vi "Utility Generate Instrument Error.vi"(8 "Error In":errorcluster, 9 "Code (0)":i32 format="%.0x", 10 "Status (F: No error)":bool, 11 "VISA Resource Name":refnum<visa-resource-name>) -> (0 "Error Out":errorcluster, 3 "VISA Resource Name Out":refnum<visa-resource-name>)   [LabVIEW 2010, in "Stanford Research 844.lvlib"]
doc: "This VI generates the error cluster with Error Code as code and chain of VI as source. The source does not include the name of this VI."
uses:
  <instrlib>/Stanford Research 844/Stanford Research 844.lvlib
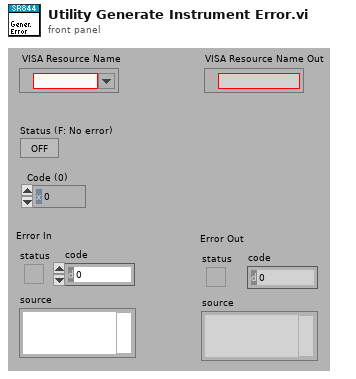
[diagram p1: front panel]
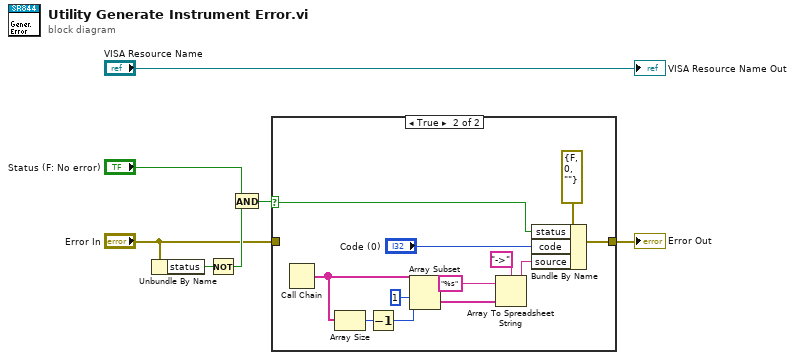
[diagram p0: block diagram]
diagram:
  n1 = Unbundle By Name("Error In") -> ("status"=w7:bool)
  n2 = Not(x=w7) -> (.not. x?=w5:bool)
  n3 = And(x="Status (F: No error)", y=w5) -> (x .and. y?=w3:bool)
  n4 = case shown="True" w3 {
    selector: w3 -> [_ w10]
    tunnel: [w8 w11] -> w6
    tunnel: "Error In" -> [w8 _]
    frame False {
    }
    frame True {
      n5 = Call Chain() -> (call chain=w19:string[])
      n6 = Array Size(array=w19) -> (size(s)=w18:i32)
      n7 = Decrement(x=w18) -> (x-1=w17:i32)
      n8 = Array Subset(array=w19, index=1 ("Array Index"), length=w17) -> (w9:string[])
      n9 = Array To Spreadsheet String(delimiter (Tab)="->", array=w9, 3:"%s" ("format string")) -> (spreadsheet string=w12:string)
      n10 = Bundle By Name(cluster=errorcluster {"status"=FALSE, "code"=0, "source"=""} ("Error Out"), "status"=w10, "code"="Code (0)", "source"=w12) -> (w11:errorcluster)
    }
  }
  "Error Out" <- w6
  "VISA Resource Name Out" <- "VISA Resource Name"
